vi "Read_DSP.vi"(8 "error in":errorcluster caption="에러 입력(에러 없음)", 10 "Byte count":u32=100, 11 "port":refnum<visa-resource-name>) -> (0 "error out":errorcluster caption="에러 출력", 2 "Data":dbl[](array[numeric]), 3 "port Out":refnum<visa-resource-name>)   [LabVIEW 2019]
panel:
  out "len":i32
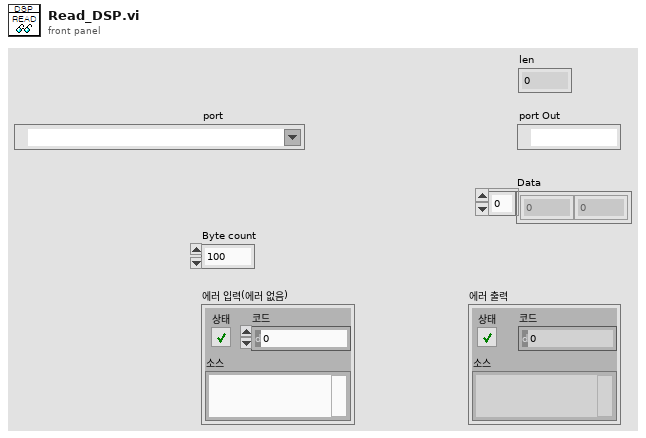
[diagram p1: front panel]
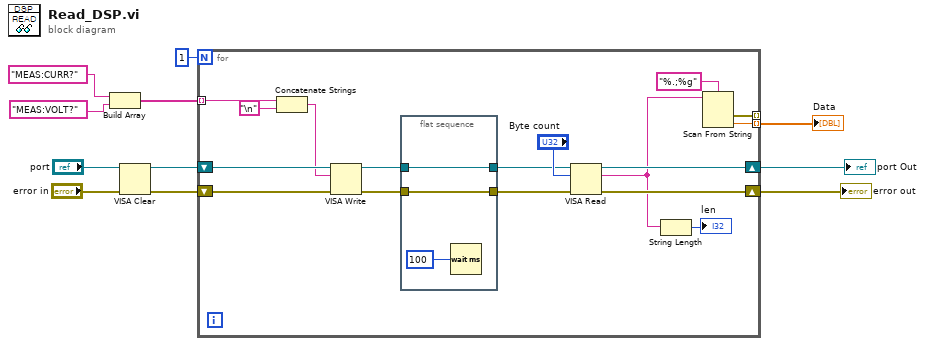
[diagram p0: block diagram]
diagram:
  n1 = Build Array("MEAS:CURR?" ("Command"), "MEAS:VOLT?" ("Command")) -> (w8:string[])
  n2 = VISA Clear(VISA resource name="port", error in (no error)="error in") -> (VISA resource name out=w6:refnum<visa-resource-name>, error out=w4:errorcluster)
  n3 = for {
    N: 1 -> [_]
    shift-right: [w26] -> w10
    shift-left: w6 -> [w28]
    shift-right: [w24] -> w9
    shift-left: w4 -> [w25]
    tunnel: w8 -> [w17] mode=indexing
    tunnel: [w15] -> w7 mode=indexing
    tunnel: [w14] -> _ mode=indexing
    n4 = Concatenate Strings(w17, "\n") -> (w19:string)
    n5 = VISA Write(VISA resource name=w28, write buffer=w19, error in (no error)=w25) -> (VISA resource name out=w23:refnum<visa-resource-name>, error out=w22:errorcluster)  [unwired: 1 out]
    n6 = flat-sequence {
      tunnel: w23 -> [w31]
      tunnel: w22 -> [w30]
      tunnel: [w31] -> w21
      tunnel: [w30] -> w20
      frame #0 {
        n7 = Wait (ms)(milliseconds to wait=u32 100 ("대기 시간 (ms)")) -> ()  [unwired: 1 out]
      }
    }
    n8 = VISA Read(VISA resource name=w21, byte count="Byte count", error in (no error)=w20) -> (VISA resource name out=w26:refnum<visa-resource-name>, read buffer=w13:string, error out=w24:errorcluster)  [unwired: 1 out]
    n9 = String Length(string=w13) -> (length=→"len":i32)
    n10 = Scan From String(format string="%.;%g", input string=w13) -> (error out=w14:errorcluster, output 1=w15:dbl)  [unwired: 3 in, 2 out]
  }
  "port Out" <- w10
  "error out" <- w9
  "Data" <- w7
